vi "gerdson.vi"   [LabVIEW 2020]
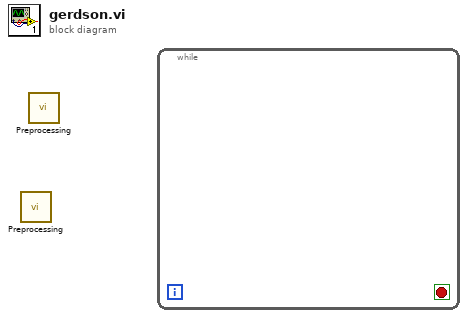
[diagram p0: block diagram]
diagram:
  n1 = call "Preprocessing.vi"() -> ()  [unwired: 4 out]
  n2 = call "Preprocessing.vi"() -> ()  [unwired: 4 out]
  n3 = while {
    stop <- _ stop-if-true
  }
